vi "FGV_RunStopTime.vi"(0 "Run Stop Time":u32, 4 "Enum":enum16{"Set", "Get"}(ring)) -> (5 "Run Stop Time (UNIX Time)":u32, 6 "Run Stop Time (UTC)":timestamp)   [LabVIEW 2018, in "feGEM DataPacker.lvlib"]
uses:
  feGEM DataPacker.lvlib
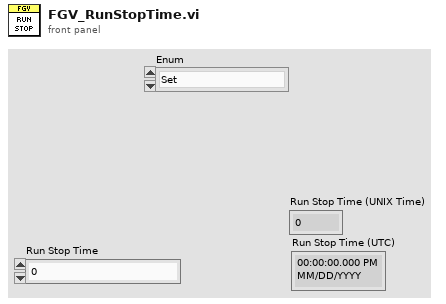
[diagram p1: front panel]
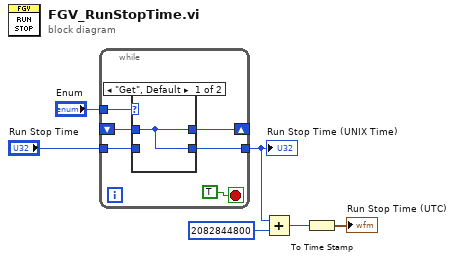
[diagram p0: block diagram]
diagram:
  n1 = while {
    shift-right: [w11] -> _
    shift-left: _ -> [w12]
    tunnel: "Run Stop Time" -> [w9]
    tunnel: [w10] -> w3
    tunnel: "Enum" -> [w8]
    stop <- TRUE stop-if-true
    n2 = case shown="\"Get\", Default" w8 {
      tunnel: [w13 w14] -> w10
      tunnel: [w13 w14] -> w11
      tunnel: w12 -> [w13 _]
      tunnel: w9 -> [_ w14]
      frame "Get", Default {
      }
      frame "Set" {
      }
    }
  }
  "Run Stop Time (UNIX Time)" <- w3
  n3 = Add(x=w3, y=u32 2082844800) -> (x+y=w1:u32)
  n4 = To Time Stamp(1:w1) -> (0:→"Run Stop Time (UTC)":timestamp)
